vi "Collect chirp parameters metadata.vi"(0 "Property Names in":string[](array[string]), 1 "Property Values in":string[](array[string]), 2 "Chirp?":bool, 3 "Chirp":T1, 5 "error in (no error)":errorcluster) -> (14 "Property names out":string[](array[string]), 15 "Property values out":string[](array[string]), 19 "error out":errorcluster)   [LabVIEW 2019, in "metadata.lvclass"]
uses:
  metadata.lvclass
  Chirp added parameters.ctl
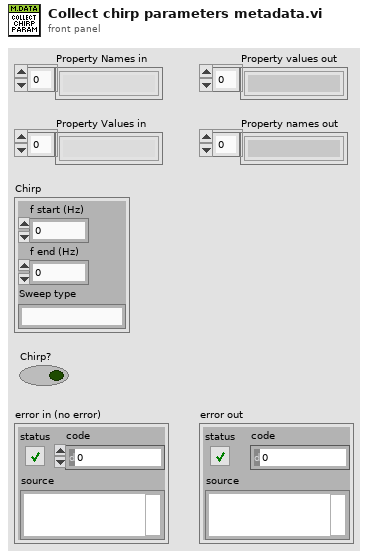
[diagram p1: front panel]
types:
  T1 = typedef "metadata.lvclass/Chirp added parameters.ctl" = cluster{"f start (Hz)":dbl, "f end (Hz)":dbl, "Sweep type":string}
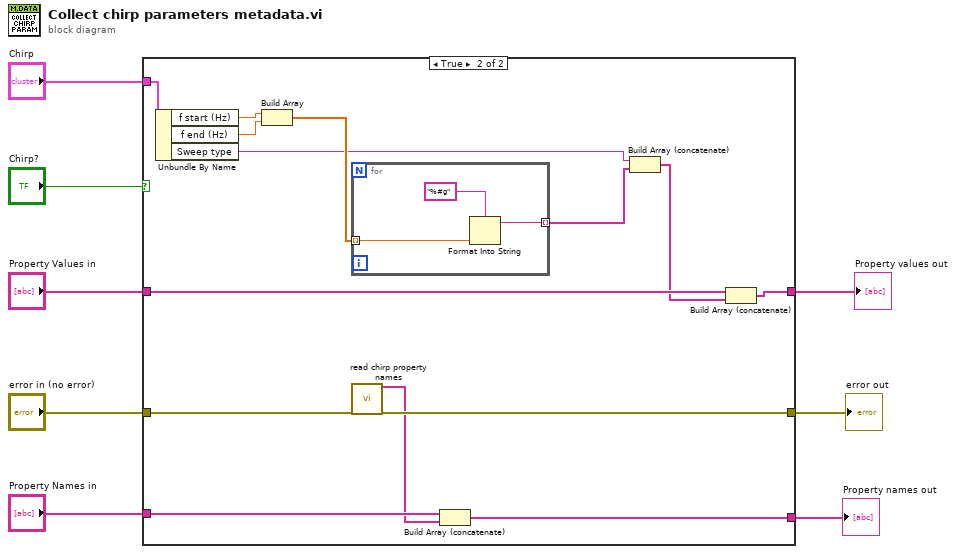
[diagram p0: block diagram]
diagram:
  n1 = case shown="True" "Chirp?" {
    tunnel: "Property Values in" -> [w10 w14]
    tunnel: [w10 w12] -> w1
    tunnel: "Property Names in" -> [w9 w23]
    tunnel: [w9 w21] -> w5
    tunnel: "error in (no error)" -> [w11 w25]
    tunnel: [w11 w24] -> w7
    tunnel: "Chirp" -> [_ w20]
    frame False {
    }
    frame True {
      n2 = Unbundle By Name(w20) -> ("f start (Hz)"=w19:dbl, "f end (Hz)"=w18:dbl, "Sweep type"=w16:string)
      n3 = Build Array(w19, w18) -> (w17:dbl[])
      n4 = for {
        tunnel: [w27] -> w15 mode=indexing
        tunnel: w17 -> [w26] mode=indexing
        n5 = Format Into String(format string="%#g", w26) -> (resulting string=w27:string)  [unwired: 2 in, 1 out]
      }
      n6 = call "read chirp property names.vi"("error in (no error)"=w25) -> ("Chirp Param"=w22:string[], "error out"=w24:errorcluster)  [unwired: 17 in]
      n7 = Build Array (concatenate)(w23, w22) -> (w21:string[])
      n8 = Build Array (concatenate)(w16, w15) -> (w13:string[])
      n9 = Build Array (concatenate)(w14, w13) -> (w12:string[])
    }
  }
  "error out" <- w7
  "Property names out" <- w5
  "Property values out" <- w1
